vi "LimeLightOutput.vi"   [LabVIEW 2019]
uses:
  9959ab12-4f3e-4c63-8bb4-e3e2fa624083.vi
  eb72db65-4b02-4b9d-91df-73159022fb0f.vi
  9959ab12-4f3e-4c63-8bb4-e3e2fa624083.vi/0e75d6ca-d504-428b-a74f-c2ed284bbcc4.vi
  eb72db65-4b02-4b9d-91df-73159022fb0f.vi/2984107b-c9c8-4aed-9355-87ed3830945a.vi
  outputs.vi
  dsdata.vi
  <vilib>/Rock Robotics/Network Tables/NT Write Value.vi
  <vilib>/Rock Robotics/Network Tables/NT Write Number.vi
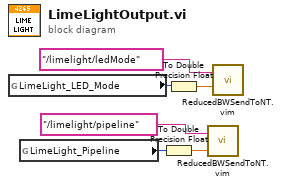
[diagram p0: block diagram]
diagram:
  n1 = global read "outputs.vi" "LimeLight_LED_Mode"() -> (w6:i64)
  n2 = global read "outputs.vi" "LimeLight_Pipeline"() -> (w5:i64)
  n3 = To Double Precision Float(number=w5) -> (double precision float=w2:dbl)
  n4 = To Double Precision Float(number=w6) -> (double precision float=w4:dbl)
  n5 = call "ReducedBWSendToNT.vim"("Value In"=w2, "NT Name"="/limelight/pipeline" ("Name")) -> ()  [unwired: 1 out]
  n6 = call "ReducedBWSendToNT.vim"("Value In"=w4, "NT Name"="/limelight/ledMode" ("Name")) -> ()  [unwired: 1 out]
